vi "main_reactor_display.vi"(5 "Storage?":refnum<vi>, 7 "Methane?":refnum<vi>, 8 "#Hydrolysis":refnum<vi>, 9 "Running?":refnum<vi>, 10 "Plant Picture":refnum<vi>, 11 "Reactor State":refnum<vi>) -> ()   [LabVIEW 2019]
uses:
  <vilib>/picture/picture.llb/imagedata.ctl
  lib/libSimulationControl/libSimulationControl.lvlib
panel:
  # "*******************************************************************\nBiogas Plant Control\n\nAuthor: Paul Zügel\nGCSC-Frankfurt am Main 2020\n\n*******************************************************************"
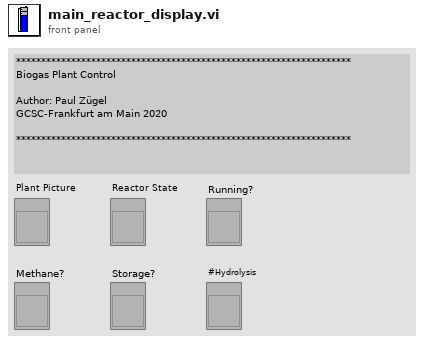
[diagram p1: front panel]
types:
  T1 = typedef "imagedata.ctl" = cluster{"image type":i32, "image depth":i32, "image":u8[], "mask":u8[], "colors":u32[], "Rectangle":cluster{"left":i16, "top":i16, "right":i16, "bottom":i16}}
  T2 = typedef "LVBoundsTypeDef.ctl" = cluster{"Width":u32, "Height":u32}
  T3 = cluster{"left":i16, "top":i16, "right":i16, "bottom":i16}
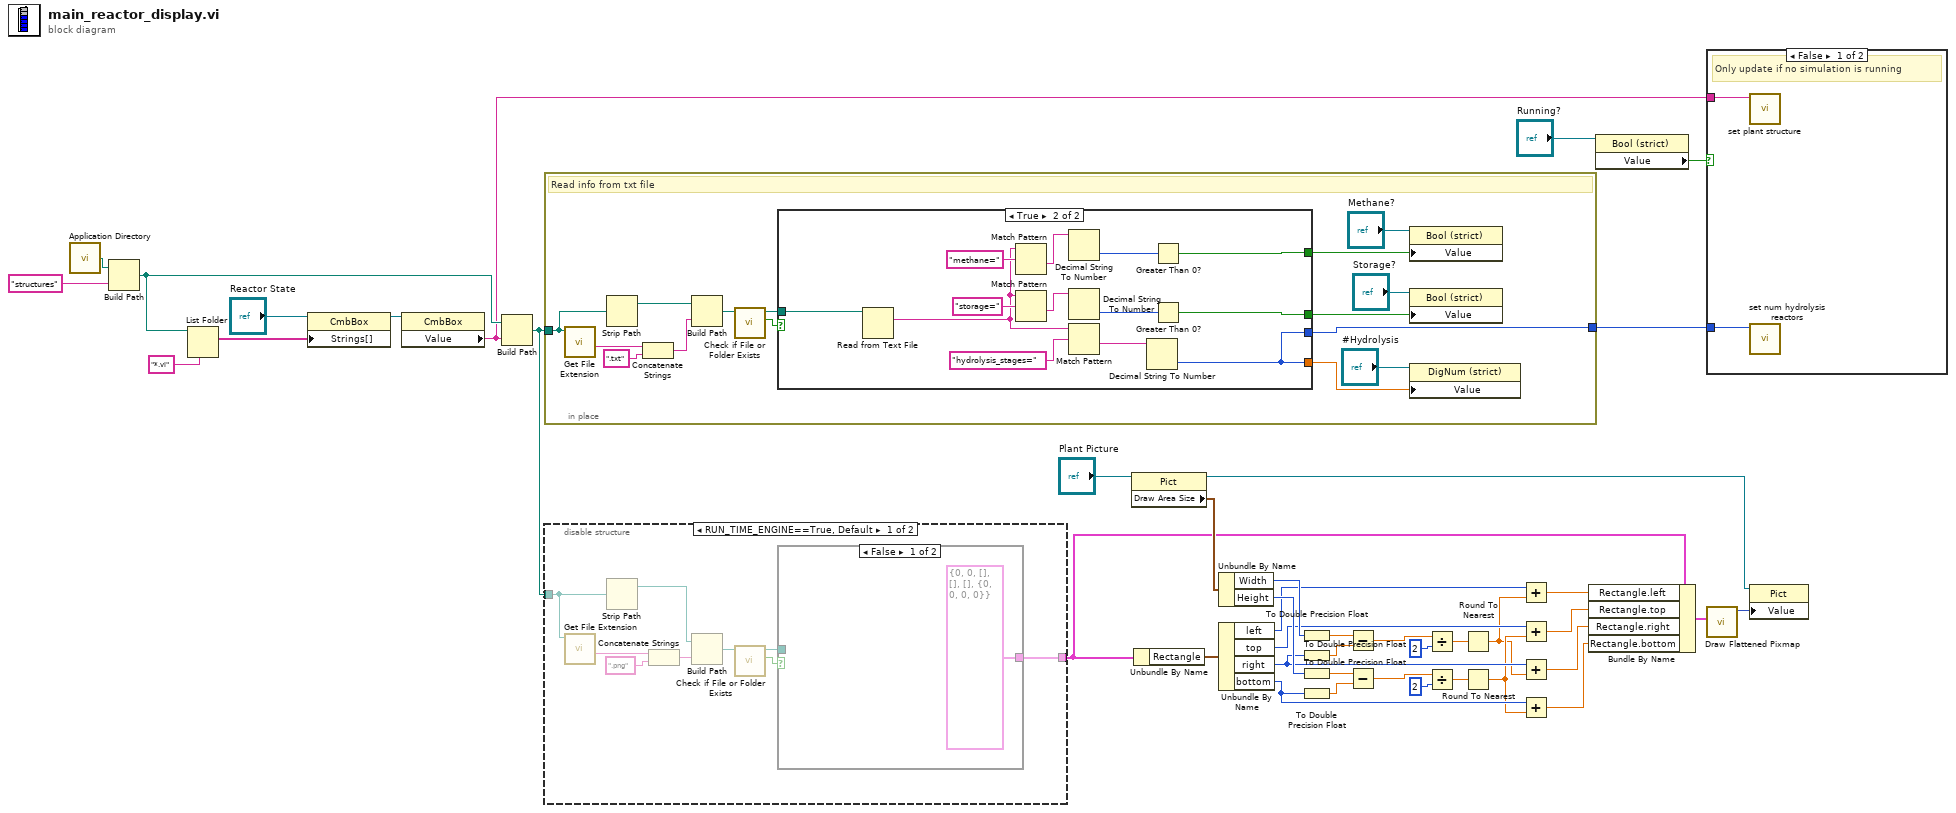
[diagram p0: block diagram]
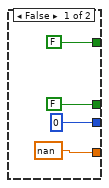
[diagram p2: hidden frame]
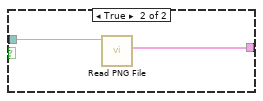
[diagram p4: hidden frame]
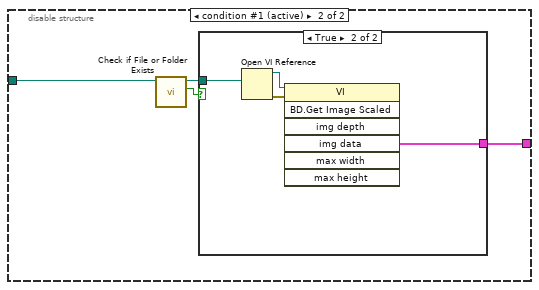
[diagram p5: hidden frame]
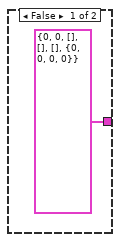
[diagram p6: hidden frame]
diagram:
  n1 = call <vilib>:"Application Directory.vi"() -> ("Application Directory"=w36:path)
  n2 = Build Path(base path=w36, name or relative path="structures") -> (appended path=w39:path)
  n3 = List Folder(path=w39, pattern="*.vi") -> (filenames=w37:string[])  [unwired: 2 in, 3 out]
  n4 = property class="CmbBox"(reference="Reactor State", "Strings[]"=w37) -> (reference out=w40:refnum<vi>)  [unwired: 1 in, 1 out]
  n5 = property class="CmbBox"(reference=w40) -> ("Value"=w3:string)  [unwired: 1 in, 2 out]
  n6 = Build Path(base path=w39, name or relative path=w3) -> (appended path=w2:path)
  n7 = in-place {
    in-place-border: w2 -> [w43]
    in-place-border: [w42] -> w1
    # "Read info from txt file"
    n8 = call <vilib>:"Get File Extension.vi"("file"=w43) -> ("filename without extension"=w44:string)  [unwired: 6 in, 4 out]
    n9 = Strip Path(path=w43) -> (stripped path=w56:path)  [unwired: 1 out]
    n10 = Concatenate Strings(w44, ".txt" ("string")) -> (w45:string)
    n11 = Build Path(base path=w56, name or relative path=w45) -> (appended path=w55:path)
    n12 = call <vilib>:"Check if File or Folder Exists.vi"("path"=w55) -> ("file or folder exists?"=w54:bool, "dup path"=w53:path)  [unwired: 8 in, 1 out]
    n13 = case shown="True" w54 {
      tunnel: w53 -> [_ w73]
      tunnel: [nan w61] -> w51
      tunnel: [FALSE ("Value") w68] -> w48
      tunnel: [FALSE ("Value") w62] -> w47
      tunnel: [0 w61] -> w42
      frame False {
      }
      frame True {
        n14 = Read from Text File(file (use dialog)=w73) -> (text=w63:string)  [unwired: 3 in, 3 out]
        n15 = Match Pattern(string=w63, regular expression="methane=") -> (after substring=w65:string)  [unwired: 1 in, 3 out]
        n16 = Match Pattern(string=w63, regular expression="storage=") -> (after substring=w69:string)  [unwired: 1 in, 3 out]
        n17 = Decimal String To Number(string=w65) -> (number=w64:i32)  [unwired: 2 in, 1 out]
        n18 = Decimal String To Number(string=w69) -> (number=w67:i32)  [unwired: 2 in, 1 out]
        n19 = Match Pattern(string=w63, regular expression="hydrolysis_stages=") -> (after substring=w71:string)  [unwired: 1 in, 3 out]
        n20 = Decimal String To Number(string=w71) -> (number=w61:i32)  [unwired: 2 in, 1 out]
        n21 = Greater Than 0?(x=w64) -> (x > 0?=w62:bool)
        n22 = Greater Than 0?(x=w67) -> (x > 0?=w68:bool)
      }
    }
    n23 = property class="Bool (strict)"(reference="Methane?", "Value"=w47) -> ()  [unwired: 1 in, 2 out]
    n24 = property class="Bool (strict)"(reference="Storage?", "Value"=w48) -> ()  [unwired: 1 in, 2 out]
    n25 = property on="Property Node" class="DigNum (strict)"(reference="#Hydrolysis", "Value"=w51) -> ()  [unwired: 1 in, 2 out]
  }
  n26 = disable-structure shown="RUN_TIME_ENGINE==True, Default" {
    disable-tunnel: w2 -> [w77 w87]
    disable-tunnel: [w74 w86] -> w9
    frame condition #0 {
      n27 = call <vilib>:"Get File Extension.vi"("file"=w77) -> ("filename without extension"=w79:string)  [unwired: 6 in, 4 out]
      n28 = Strip Path(path=w77) -> (stripped path=w81:path)  [unwired: 1 out]
      n29 = Concatenate Strings(w79, ".png" ("string")) -> (w82:string)
      n30 = Build Path(base path=w81, name or relative path=w82) -> (appended path=w80:path)
      n31 = call <vilib>:"Check if File or Folder Exists.vi"("path"=w80) -> ("file or folder exists?"=w76:bool, "dup path"=w75:path)  [unwired: 8 in, 1 out]
      n32 = case shown="False" w76 {
        tunnel: w75 -> [_ w85]
        tunnel: [T1 {"image type"=0, "image depth"=0, "image"=[], "mask"=[], "colors"=[], "Rectangle"={"left"=0, "top"=0, "right"=0, "bottom"=0}} ("image data") w84] -> w74
        frame False {
        }
        frame True {
          n33 = call <vilib>:"Read PNG File.vi"("path to PNG file"=w85) -> ("image data"=w84:T1)  [unwired: 8 in, 2 out]
        }
      }
    }
    frame condition #1 (active) {
      n34 = call <vilib>:"Check if File or Folder Exists.vi"("path"=w87) -> ("file or folder exists?"=w88:bool, "dup path"=w89:path)  [unwired: 8 in, 1 out]
      n35 = case shown="True" w88 {
        tunnel: w89 -> [_ w92]
        tunnel: [T1 {"image type"=0, "image depth"=0, "image"=[], "mask"=[], "colors"=[], "Rectangle"={"left"=0, "top"=0, "right"=0, "bottom"=0}} ("img data") w91] -> w86
        frame False {
        }
        frame True {
          n36 = Open VI Reference(vi path=w92) -> (vi reference=w94:refnum<vi>, error out=w93:errorcluster)  [unwired: 5 in]
          n37 = invoke class="VI" method="BD.Get Image Scaled"(reference=w94, error in=w93) -> ("img data"=w91:T1)  [unwired: 5 in, 6 out]
        }
      }
    }
  }
  n38 = property class="Pict"(reference="Plant Picture") -> (reference out=w7:refnum<vi>, "Draw Area Size"=w12:T2)  [unwired: 1 in, 1 out]
  n39 = Unbundle By Name(w9) -> ("Rectangle"=w14:T3)
  n40 = Unbundle By Name(w12) -> ("Width"=w29:u32, "Height"=w33:u32)
  n41 = Unbundle By Name(w14) -> ("left"=w15:i16, "top"=w25:i16, "right"=w27:i16, "bottom"=w31:i16)
  n42 = To Double Precision Float(number=w29) -> (double precision float=w28:dbl)
  n43 = To Double Precision Float(number=w27) -> (double precision float=w26:dbl)
  n44 = To Double Precision Float(number=w33) -> (double precision float=w32:dbl)
  n45 = To Double Precision Float(number=w31) -> (double precision float=w30:dbl)
  n46 = Subtract(x=w28, y=w26) -> (x-y=w13:dbl)
  n47 = Subtract(x=w32, y=w30) -> (x-y=w21:dbl)
  n48 = Divide(x=w13, y=u32 2) -> (x/y=w18:dbl)
  n49 = Divide(x=w21, y=u32 2) -> (x/y=w20:dbl)
  n50 = Round To Nearest(number=w18) -> (nearest integer value=w19:dbl)
  n51 = Round To Nearest(number=w20) -> (nearest integer value=w22:dbl)
  n52 = Add(x=w15, y=w19) -> (x+y=w16:dbl)
  n53 = Add(x=w25, y=w22) -> (x+y=w23:dbl)
  n54 = Add(x=w27, y=w19) -> (x+y=w17:dbl)
  n55 = Add(x=w31, y=w22) -> (x+y=w24:dbl)
  n56 = Bundle By Name(cluster=w9, "Rectangle.left"=w16, "Rectangle.top"=w23, "Rectangle.right"=w17, "Rectangle.bottom"=w24) -> (w8:T1)
  n57 = property class="Bool (strict)"(reference="Running?") -> ("Value"=w4:bool)  [unwired: 1 in, 2 out]
  n58 = case shown="False" w4 {
    tunnel: w3 -> [w96 _]
    tunnel: w1 -> [w95 _]
    frame False {
      # "Only update if no simulation is running"
      n59 = call "set plant structure.vi"("structure"=w96) -> ()  [unwired: 10 in, 1 out]
      n60 = call "set num hydrolysis reactors.vi"("num"=w95) -> ()  [unwired: 10 in, 1 out]
    }
    frame True {
    }
  }
  n61 = call <vilib>:"Draw Flattened Pixmap.vi"("image data"=w8) -> ("new picture"=w34:picture)  [unwired: 8 in]
  n62 = property class="Pict"(reference=w7, "Value"=w34) -> ()  [unwired: 1 in, 2 out]
